vi "Configure.vi"(8 "error in (no error)":errorcluster, 11 "Waveform in":refnum<class "Waveform.lvclass">) -> (0 "error out":errorcluster, 2 "cancelled?":bool, 3 "Waveform out":refnum<class "Waveform.lvclass">)   [LabVIEW 2012, in "Waveform.lvclass"]
doc: "The configure method configures the details for the RabbitMQ connection, the observers and the mapping script.\n\nIn the derived class, make a call to the parent for setting these parameters."
uses:
  Waveform.lvclass
  <vilib>/Utility/miscctls.llb/LVPointTypeDef.ctl
  Waveform.lvclass/Waveform.ctl
  <vilib>/Distrio/Murmex/Murmex/Murmex.lvclass
panel:
  in  "button::cancel":bool
  in  "button::ok":bool
  in  "button::configure murmex":bool
  in  "Tab Control":T1(tab)
  in  "Output Terminal C2":tag="/Dev1/PFI12" caption="Output Terminal"
  in  "C2":tag="Dev1/ctr1" caption="Counter"
  in  "Duty cycle 2":dbl caption="Duty cycle"
  in  "Output Terminal C1":tag="/Dev1/PFI12" caption="Output Terminal"
  in  "C1":tag="Dev1/ctr0" caption="Counter"
  in  "PI stage trigger":tag
  in  "% camera frame rate":dbl
  in  "Duty cycle":dbl
  in  "PC Physical Channel":tag="Dev1/ao0" caption="Physical Channel"
  in  "min Voltage 3":dbl caption="min Voltage"
  in  "max Voltage 3":dbl caption="max Voltage"
  in  "Galvos Physical Channels":tag="Dev1/ao0" caption="Physical Channel"
  in  "min Voltage":dbl
  in  "max Voltage":dbl
  in  "Shutter line":tag="Dev1/port0/line0:7"
  in  "Autofocus":string
  in  "Tomo":string
  in  "Stack":string
  in  "LineCCD":string
  in  "target component ID":string
  in  "AddRelayTarget":bool
  in  "RemoveRelayTarget":bool
  in  "relay start/stop to...":i32(listbox)
  in  "Orca- Master":string
  in  "Orca- Slave":string
  in  "Cascade":string
  # "RabbitMQ parameters"
  # "Window position"
  # "Sends a setting or configuration value to an observer, e.g. observer.parameter=settingsname;"
  # "Clock for AO channels"
  # "Frame trigger"
  # "Galvo 1&2"
  # "Pockels Cell"
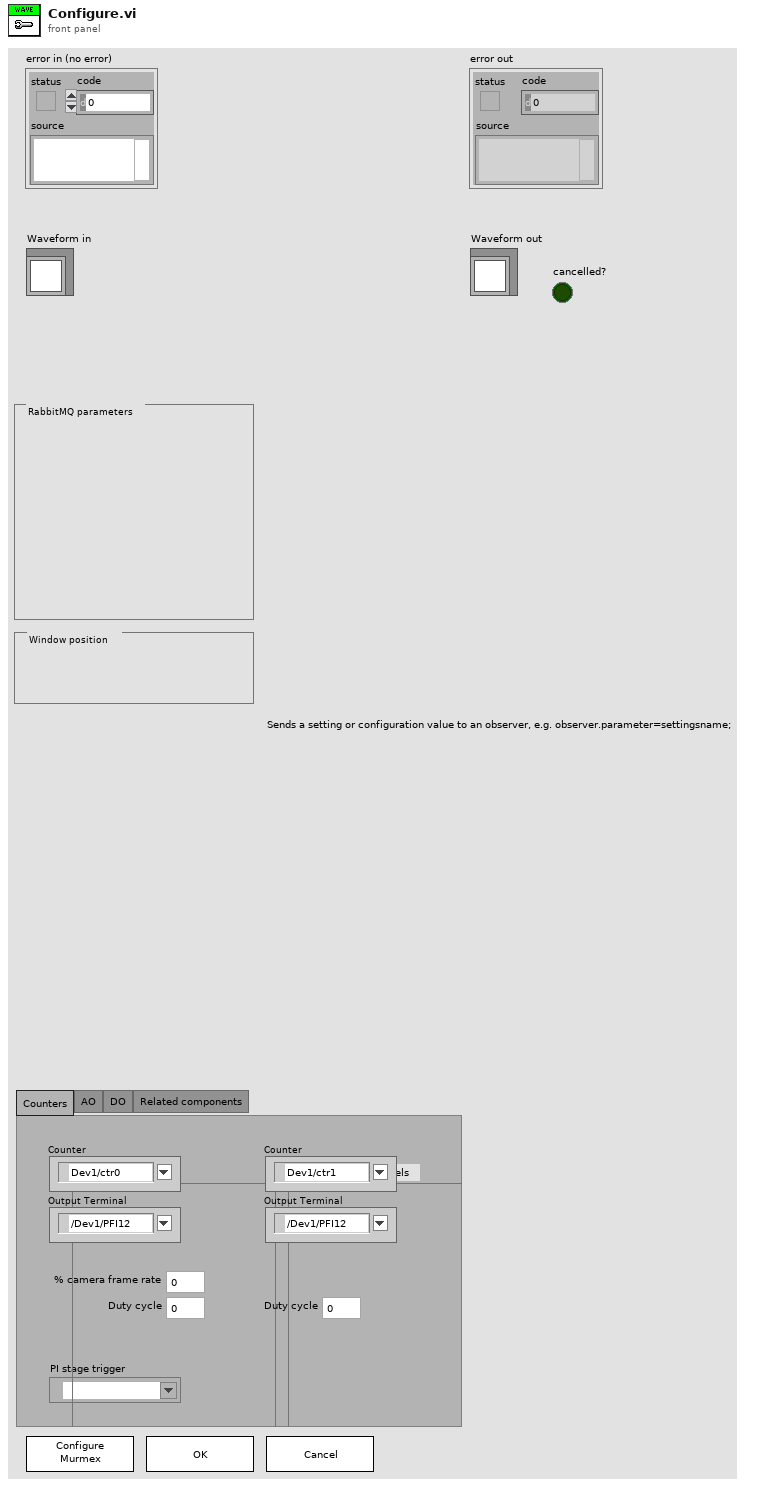
[diagram p1: front panel]
types:
  T1 = enum32{"Counters", "AO", "DO", "Related components"}
  T2 = typedef "LVPointTypeDef.ctl" = cluster{"Horizontal":i16, "Vertical":i16}
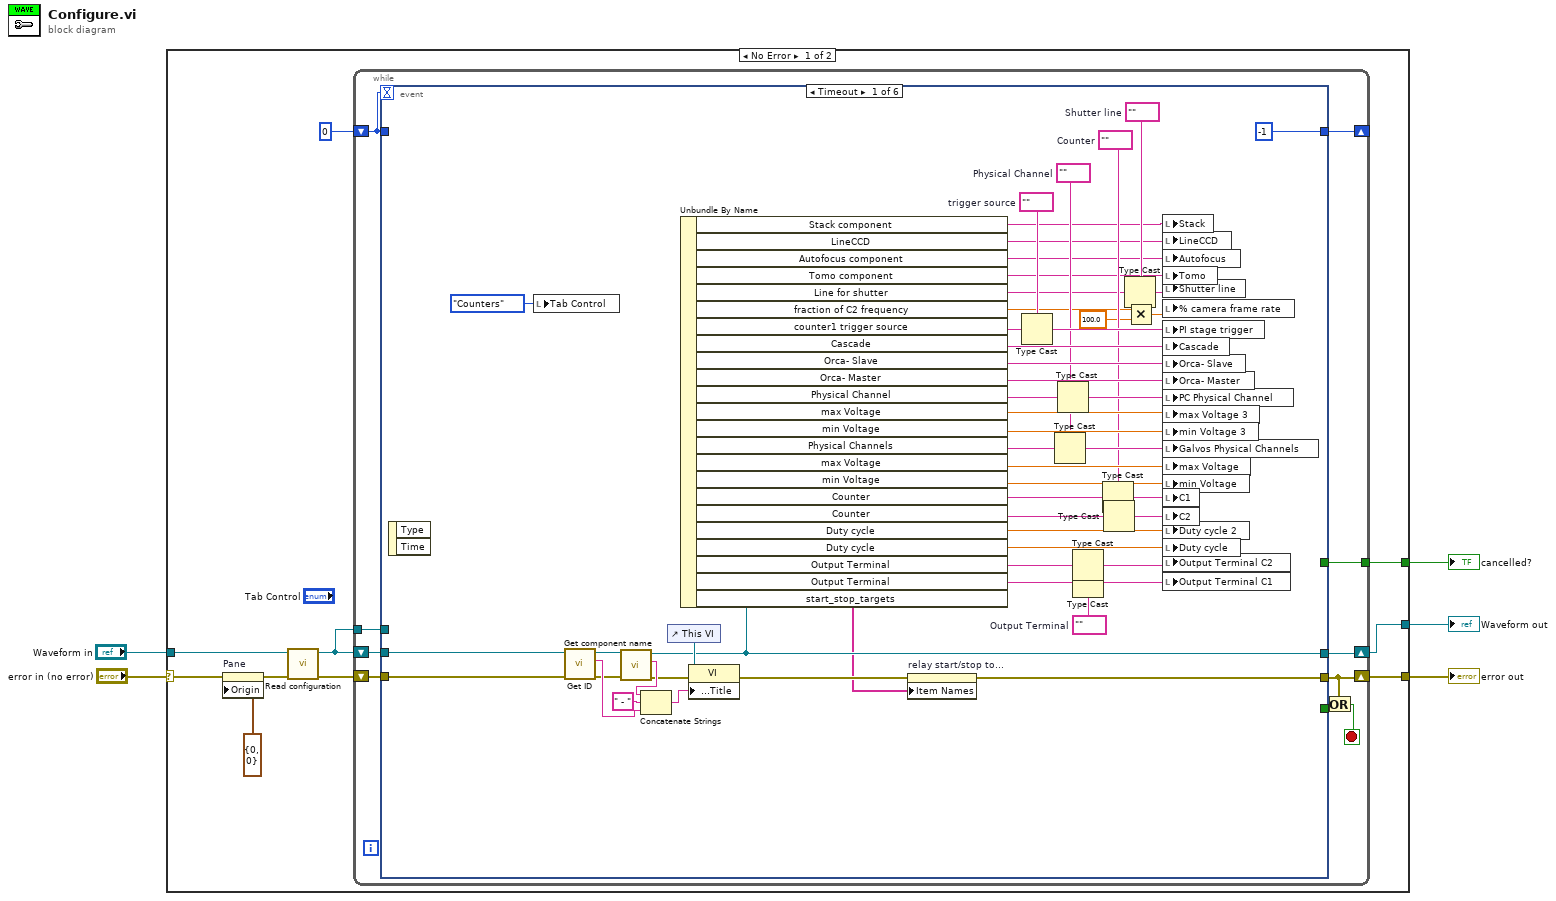
[diagram p0: block diagram]
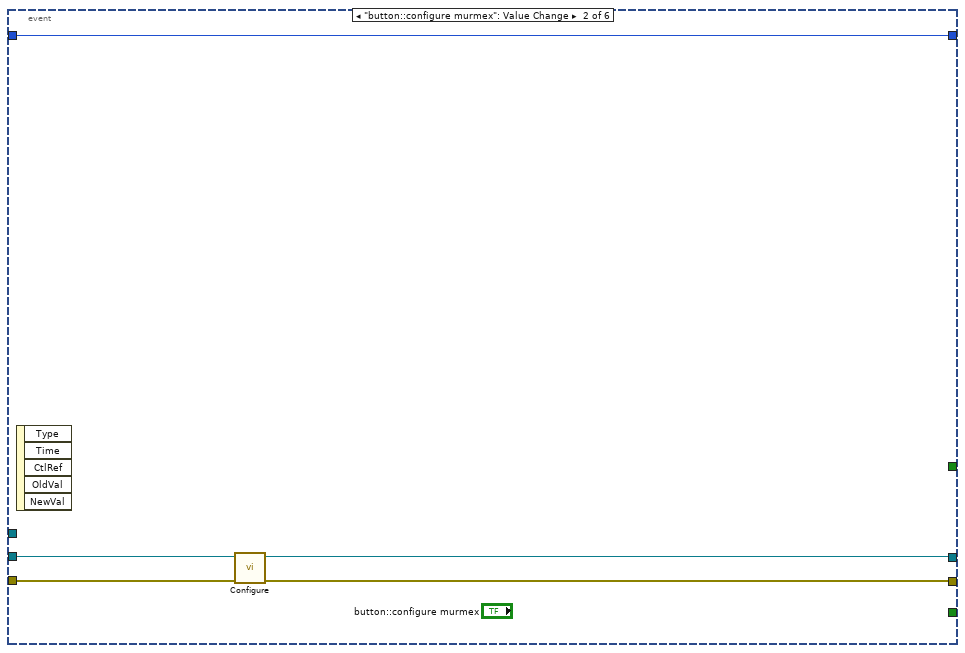
[diagram p2: hidden frame]
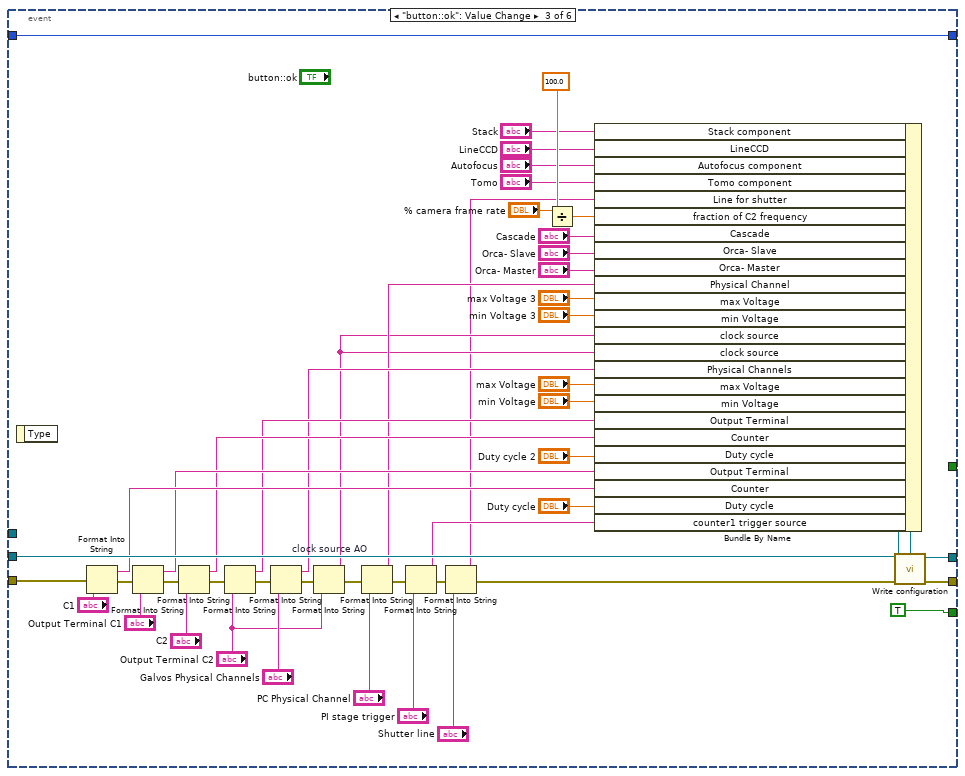
[diagram p3: hidden frame]
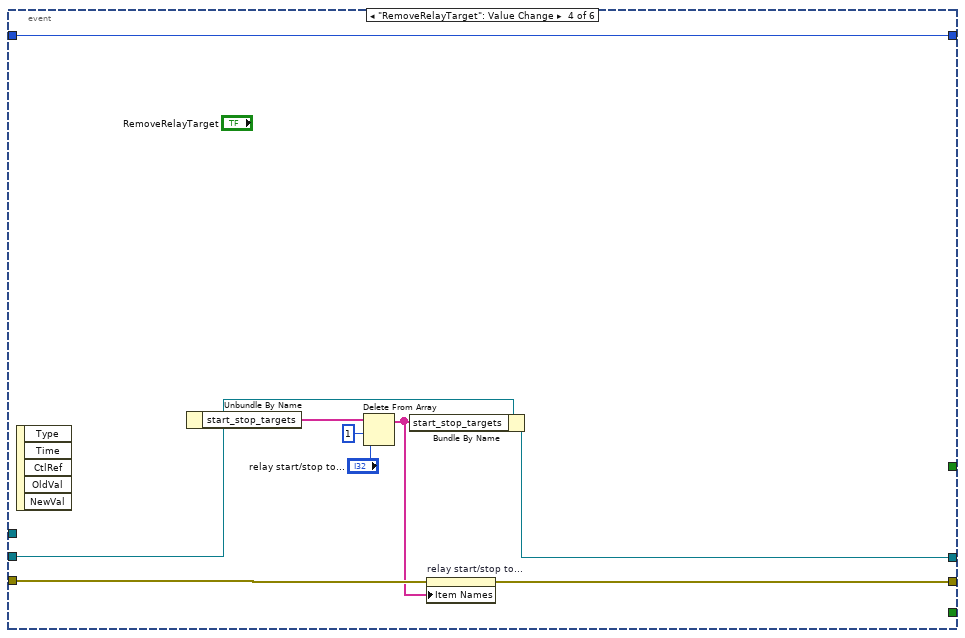
[diagram p4: hidden frame]
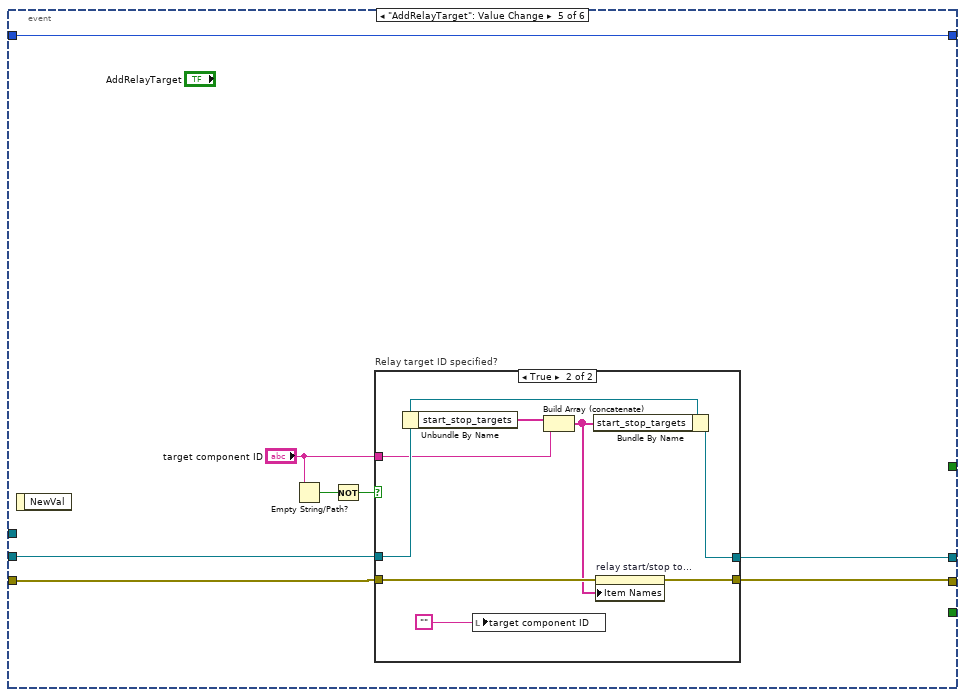
[diagram p5: hidden frame]
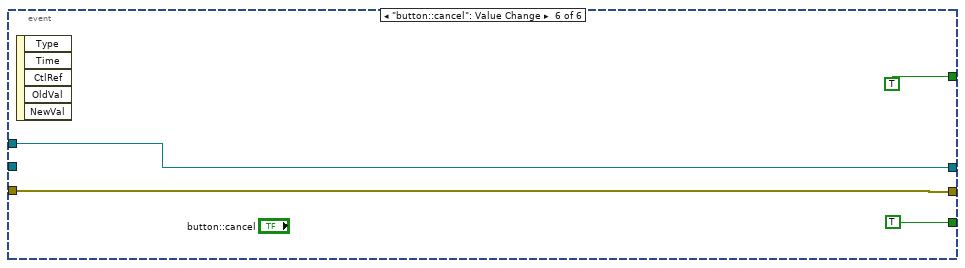
[diagram p7: hidden frame]
diagram:
  n1 = case shown="No Error" "error in (no error)" {
    selector: "error in (no error)" -> [w14 w165]
    tunnel: "Waveform in" -> [w12 w164]
    tunnel: [w8 w165] -> w3
    tunnel: [w7 w164] -> w2
    tunnel: [w6 _] -> w1
    frame No Error {
      n2 = property on="Pane" class="Pane"(error in=w14, "Origin"=T2 {"Horizontal"=0, "Vertical"=0}) -> (error out=w13:errorcluster)  [unwired: 1 in, 1 out]
      n3 = call <vilib>:"Read configuration.vi"("error in (no error)"=w13, "Murmex in"=w12) -> ("error out"=w11:errorcluster, "Murmex out"=w10:refnum<class "Waveform.lvclass">)  [unwired: 7 in, 1 out]
      n4 = while {
        shift-right: [w19] -> w8
        shift-left: w11 -> [w25]
        shift-right: [w21] -> w7
        shift-left: w10 -> [w23]
        tunnel: w10 -> [w24]
        shift-right: [w20] -> _
        shift-left: 0 -> [w22]
        tunnel: [w16] -> w6
        stop <- w18 stop-if-true
        n5 = event shown="[0] Timeout" {
          selector: _ -> [_ _ _ _ _ _]
          dyn-events: _ -> [_ _ _ _ _ _]
          timeout: w22 -> [_ _ _ _ _ _]
          tunnel: w25 -> [w78 w83 w118 w135 w145 w163]
          tunnel: w24 -> [_ _ _ _ _ w162]
          tunnel: w23 -> [w77 w80 w119 w137 w148 _]
          tunnel: w22 -> [_ w81 w120 w141 w149 _]
          tunnel: [w38 w82 w131 w134 w144 w163] -> w19
          tunnel: [w68 w79 w132 w136 w147 w162] -> w21
          tunnel: [-1 w81 w120 w141 w149 _] -> w20
          tunnel: [_ _ TRUE _ _ TRUE ("force loading?")] -> w17
          tunnel: [_ _ _ _ _ TRUE ("force loading?")] -> w16
          event Timeout {
            w31 = tag ""  # Shutter line
            w40 = tag ""  # Counter
            w42 = tag ""  # trigger source
            w45 = tag ""  # Output Terminal
            w41 = tag ""  # Physical Channel
            n6 = event-data() -> ()  [unwired: 1 in, 2 out]
            n7 = local write "Tab Control"(T1."Counters" ("Tab Control")) -> ()
            n8 = call <vilib>:"Get ID.vi"("error in (no error)"=w78, "Murmex in"=w77) -> ("error out"=w72:errorcluster, "component id"=w75:string, "Murmex out"=w73:refnum<class "Waveform.lvclass">)  [unwired: 7 in]
            n9 = call <vilib>:"Get component name.vi"("error in (no error)"=w72, "Murmex in"=w73) -> ("error out"=w70:errorcluster, "component name"=w74:string, "Murmex out"=w68:refnum<class "Waveform.lvclass">)  [unwired: 7 in]
            n10 = Concatenate Strings(w74, " - " ("string"), w75) -> (w69:string)
            n11 = control-ref of="This VI"() -> (w71:refnum<vi>)
            n12 = Unbundle By Name(w68) -> ("Stack component"=w27:string, "LineCCD"=w28:string, "Autofocus component"=w29:string, "Tomo component"=w30:string, "Line for shutter"=w33:string, "fraction of C2 frequency"=w36:dbl, "counter1 trigger source"=w44:string, "Cascade"=w58:string, "Orca- Slave"=w59:string, "Orca- Master"=w60:string, "Physical Channel"=w57:string, "max Voltage"=w61:dbl, "min Voltage"=w62:dbl, "Physical Channels"=w54:string, "max Voltage"=w63:dbl, "min Voltage"=w64:dbl, "Counter"=w50:string, "Counter"=w52:string, "Duty cycle"=w65:dbl, "Duty cycle"=w66:dbl, "Output Terminal"=w48:string, "Output Terminal"=w46:string, "start_stop_targets"=w37:string[])
            n13 = property class="VI"(reference=w71, error in=w70, "Front Panel.Title"=w69) -> (error out=w39:errorcluster)  [unwired: 1 out]
            n14 = property on="relay start/stop to..." class="LstBox (strict)"(error in=w39, "Item Names"=w37) -> (error out=w38:errorcluster)  [unwired: 1 in, 1 out]
            n15 = Type Cast(type=w42, x=w44) -> (*(type *) &x=w43:tag)
            n16 = Type Cast(type=w41, x=w54) -> (*(type *) &x=w55:tag)
            n17 = Type Cast(type=w41, x=w57) -> (*(type *) &x=w56:tag)
            n18 = Type Cast(type=w45, x=w48) -> (*(type *) &x=w49:tag)
            n19 = Type Cast(type=w45, x=w46) -> (*(type *) &x=w47:tag)
            n20 = Type Cast(type=w40, x=w50) -> (*(type *) &x=w51:tag)
            n21 = Type Cast(type=w40, x=w52) -> (*(type *) &x=w53:tag)
            n22 = Type Cast(type=w31, x=w33) -> (*(type *) &x=w32:tag)
            n23 = Multiply(x=w36, y=100.0) -> (x*y=w35:dbl)
            n24 = local write "Stack"(w27) -> ()
            n25 = local write "LineCCD"(w28) -> ()
            n26 = local write "Autofocus"(w29) -> ()
            n27 = local write "Tomo"(w30) -> ()
            n28 = local write "Shutter line"(w32) -> ()
            n29 = local write "% camera frame rate"(w35) -> ()
            n30 = local write "PI stage trigger"(w43) -> ()
            n31 = local write "Cascade"(w58) -> ()
            n32 = local write "Orca- Slave"(w59) -> ()
            n33 = local write "Orca- Master"(w60) -> ()
            n34 = local write "PC Physical Channel"(w56) -> ()
            n35 = local write "max Voltage 3"(w61) -> ()
            n36 = local write "min Voltage 3"(w62) -> ()
            n37 = local write "Galvos Physical Channels"(w55) -> ()
            n38 = local write "max Voltage"(w63) -> ()
            n39 = local write "min Voltage"(w64) -> ()
            n40 = local write "C1"(w51) -> ()
            n41 = local write "C2"(w53) -> ()
            n42 = local write "Duty cycle 2"(w65) -> ()
            n43 = local write "Duty cycle"(w66) -> ()
            n44 = local write "Output Terminal C2"(w49) -> ()
            n45 = local write "Output Terminal C1"(w47) -> ()
          }
          event "button::configure murmex": Value Change {
            n46 = event-data() -> ()  [unwired: 1 in, 5 out]
            n47 = call-parent "Configure.vi"("error in (no error)"=w83, "Murmex in"=w80) -> ("error out"=w82:errorcluster, "Murmex out"=w79:refnum<class "Waveform.lvclass">)  [unwired: 7 in, 1 out]
          }
          event "button::ok": Value Change {
            n48 = event-data() -> ()  [unwired: 1 in, 1 out]
            n49 = Format Into String(error in=w118, "C1") -> (resulting string=w107:string, error out=w116:errorcluster)  [unwired: 2 in]
            n50 = Format Into String(error in=w116, "Output Terminal C1") -> (resulting string=w106:string, error out=w114:errorcluster)  [unwired: 2 in]
            n51 = Format Into String(error in=w114, "C2") -> (resulting string=w105:string, error out=w112:errorcluster)  [unwired: 2 in]
            n52 = Format Into String(error in=w112, "Output Terminal C2") -> (resulting string=w104:string, error out=w111:errorcluster)  [unwired: 2 in]
            n53 = Format Into String(error in=w111, "Galvos Physical Channels") -> (resulting string=w103:string, error out=w109:errorcluster)  [unwired: 2 in]
            n54 = Format Into String "clock source AO"(error in=w109, "Output Terminal C2") -> (resulting string=w101:string, error out=w96:errorcluster)  [unwired: 2 in]
            n55 = Format Into String(error in=w96, "PC Physical Channel") -> (resulting string=w102:string, error out=w99:errorcluster)  [unwired: 2 in]
            n56 = Format Into String(error in=w99, "PI stage trigger") -> (resulting string=w97:string, error out=w91:errorcluster)  [unwired: 2 in]
            n57 = Format Into String(error in=w91, "Shutter line") -> (resulting string=w88:string, error out=w90:errorcluster)  [unwired: 2 in]
            n58 = Divide(x="% camera frame rate", y=100.0) -> (x/y=w92:dbl)
            n59 = Bundle By Name(cluster=w119, "Stack component"="Stack", "LineCCD"="LineCCD", "Autofocus component"="Autofocus", "Tomo component"="Tomo", "Line for shutter"=w88, "fraction of C2 frequency"=w92, "Cascade"="Cascade", "Orca- Slave"="Orca- Slave", "Orca- Master"="Orca- Master", "Physical Channel"=w102, "max Voltage"="max Voltage 3", "min Voltage"="min Voltage 3", "clock source"=w101, "clock source"=w101, "Physical Channels"=w103, "max Voltage"="max Voltage", "min Voltage"="min Voltage", "Output Terminal"=w104, "Counter"=w105, "Duty cycle"="Duty cycle 2", "Output Terminal"=w106, "Counter"=w107, "Duty cycle"="Duty cycle", "counter1 trigger source"=w97) -> (w130:refnum<class "Waveform.lvclass">)
            n60 = call <vilib>:"Write configuration.vi"("error in (no error)"=w90, "Murmex in"=w130) -> ("error out"=w131:errorcluster, "Murmex out"=w132:refnum<class "Waveform.lvclass">)  [unwired: 8 in]
          }
          event "RemoveRelayTarget": Value Change {
            n61 = event-data() -> ()  [unwired: 1 in, 5 out]
            n62 = Unbundle By Name(w137) -> ("start_stop_targets"=w140:string[])
            n63 = Delete From Array(array=w140, length=1, index="relay start/stop to...") -> (array with subset deleted=w133:string[])  [unwired: 1 out]
            n64 = Bundle By Name(cluster=w137, "start_stop_targets"=w133) -> (w136:refnum<class "Waveform.lvclass">)
            n65 = property on="relay start/stop to..." class="LstBox (strict)"(error in=w135, "Item Names"=w133) -> (error out=w134:errorcluster)  [unwired: 1 in, 1 out]
          }
          event "AddRelayTarget": Value Change {
            n66 = event-data() -> ()  [unwired: 1 in, 1 out]
            n67 = Empty String/Path?(string/path="target component ID") -> (empty?=w143:bool)
            n68 = Not(x=w143) -> (.not. x?=w142:bool)
            n69 = case "Relay target ID specified?" shown="True" w142 {
              tunnel: w148 -> [w151 w159]
              tunnel: [w151 w158] -> w147
              tunnel: "target component ID" -> [_ w156]
              tunnel: w145 -> [w150 w154]
              tunnel: [w150 w153] -> w144
              frame False {
              }
              frame True {
                n70 = Unbundle By Name(w159) -> ("start_stop_targets"=w157:string[])
                n71 = local write "target component ID"("") -> ()
                n72 = Build Array (concatenate)(w157, w156) -> (w152:string[])
                n73 = Bundle By Name(cluster=w159, "start_stop_targets"=w152) -> (w158:refnum<class "Waveform.lvclass">)
                n74 = property on="relay start/stop to..." class="LstBox (strict)"(error in=w154, "Item Names"=w152) -> (error out=w153:errorcluster)  [unwired: 1 in, 1 out]
              }
            }
          }
          event "button::cancel": Value Change {
            n75 = event-data() -> ()  [unwired: 1 in, 5 out]
          }
        }
        n76 = Or(x=w19, y=w17) -> (x .or. y?=w18:bool)
      }
    }
    frame Error {
    }
  }
  "error out" <- w3
  "Waveform out" <- w2
  "cancelled?" <- w1
